vi "NI 9230 Getting Started (FPGA).vi"() -> ()   [LabVIEW 2021]
doc: "This VI acquires an arbitrary number of samples from each channel of the NI 9232 and places the acquired data into a DMA FIFO. The Input Configuration and Data Rate are configurable at run time."
uses:
  <vilib>/LabVIEW Targets/FPGA/cRIO/shared/nicrio_ModuleControls/nicrio_cRIO-9232_ConfigModeRing.ctl
  <vilib>/LabVIEW Targets/FPGA/cRIO/shared/nicrio_ModuleControls/nicrio_cRIO-9230_DataRatesRing2.ctl
  <vilib>/rvi/Emulation/niFpgaGetClockAttributes.vi
  <vilib>/rvi/Emulation/niFpgaSctlEmulationGetInTimedLoop.vi
  <vilib>/rvi/Emulation/niFpgaEmulationReportErrorSimple.vi
  <vilib>/rvi/eio/common/nirviEmuTemplatePropertySet_errors.vi
  <vilib>/rvi/eio/common/nirviEmuTemplateMethod_errors.vi
  <vilib>/rvi/interface/RandomDataEmulation/niFpgaRandomDataHandleErrors.vi
  <vilib>/rvi/Emulation/niFpgaCriticalErrorInLSC.vi
  <vilib>/eio/EIOPropertyNode/EIOPropertyNode.xnode
  <vilib>/eio/EIONode/EIONode.xnode
  <vilib>/rvi/DataTransferAndStorage/Container/XNode/niFpgaContainer.xnode
  <vilib>/rvi/interface/RandomDataEmulation/nirviRandomDataFpgaReadWriteTemplate.vi
  <vilib>/eio/EIOMethodNode/EIOMethodNode.xnode
  <vilib>/rvi/eio/common/nirviEmuTemplatePropertyGet_errors.vi
  <vilib>/rvi/eio/common/nirviEmuTemplatePropertyGet_noerrors.vi
  <vilib>/rvi/eio/common/nirviEmuTemplatePropertySet_noerrors.vi
panel:
  in  "Input Configuration 1":T1 items=["AC Coupled", "DC Coupled", "IEPE AC Coupled"]
  in  "Input Configuration 0":T1 items=["AC Coupled", "DC Coupled", "IEPE AC Coupled"]
  in  "Data Rate":T2=10 items=["12.800 kS/s (NI 9230)"=10, "11.378 kS/s (NI 9230)"=36, "10.240 kS/s (NI 9230)"=21, "9.309 kS/s (NI 9230)"=44, "8.533 kS/s (NI 9230)"=14, "7.877 kS/s (NI 9230)"=52, "7.314 kS/s (NI 9230)"=29, "6.827 kS/s (NI 9230)"=60, "6.400 kS/s (NI 9230)"=18, "6.024 kS/s (NI 9230)"=68, "5.689 kS/s (NI 9230)"=37, "5.389 kS/s (NI 9230)"=76, "5.120 kS/s (NI 9230)"=22, "4.876 kS/s (NI 9230)"=84, "4.655 kS/s (NI 9230)"=45, "4.452 kS/s (NI 9230)"=92, "4.267 kS/s (NI 9230)"=26, "4.096 kS/s (NI 9230)"=100, "3.938 kS/s (NI 9230)"=53, "3.657 kS/s (NI 9230)"=30, "3.413 kS/s (NI 9230)"=61, "3.200 kS/s (NI 9230)"=34, "3.012 kS/s (NI 9230)"=69, "2.844 kS/s (NI 9230)"=38, "2.695 kS/s (NI 9230)"=77, "2.560 kS/s (NI 9230)"=42, "2.438 kS/s (NI 9230)"=85, "2.327 kS/s (NI 9230)"=46, "2.226 kS/s (NI 9230)"=93, "2.133 kS/s (NI 9230)"=50, "2.048 kS/s (NI 9230)"=101, "1.969 kS/s (NI 9230)"=54, "1.829 kS/s (NI 9230)"=58, "1.707 kS/s (NI 9230)"=62, "1.600 kS/s (NI 9230)"=66, "1.506 kS/s (NI 9230)"=70, "1.422 kS/s (NI 9230)"=74, "1.347 kS/s (NI 9230)"=78, "1.280 kS/s (NI 9230)"=82, "1.219 kS/s (NI 9230)"=86, "1.164 kS/s (NI 9230)"=90, "1.113 kS/s (NI 9230)"=94, "1.067 kS/s (NI 9230)"=98, "1.024 kS/s (NI 9230)"=102, "0.985 kS/s (NI 9230)"=106]
  out "Error Out":errorcluster
  out "Short Circuit":bool[](array[boolean])
  out "Open Loop":bool[](array[boolean])
  in  "Input Configuration 2":T1 items=["AC Coupled", "DC Coupled", "IEPE AC Coupled"]
  out "Data FIFO Full":bool
  # "Overview: Demonstrates how to acquire data from the NI 9230\nRequirements: LabVIEW Full Development System, LV FPGA, and NI RIO\nInstructions: \n1. Run NI 9230 Getting Started (Host).vi"
  # "Input Parameters"
  # "Output Parameters"
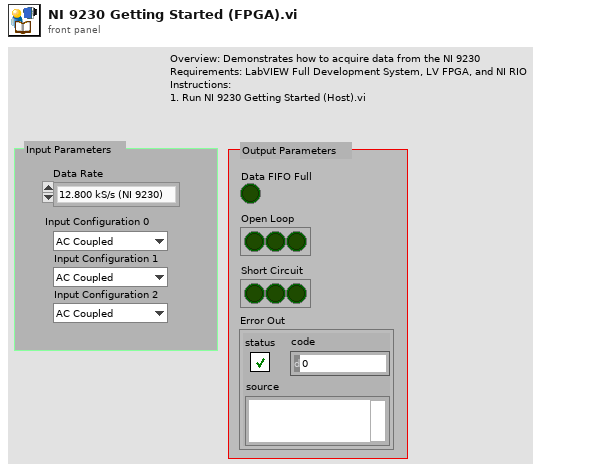
[diagram p1: front panel]
types:
  T1 = typedef "nicrio_cRIO-9232_ConfigModeRing.ctl" = u8
  T2 = typedef "nicrio_cRIO-9230_DataRatesRing2.ctl" = u8
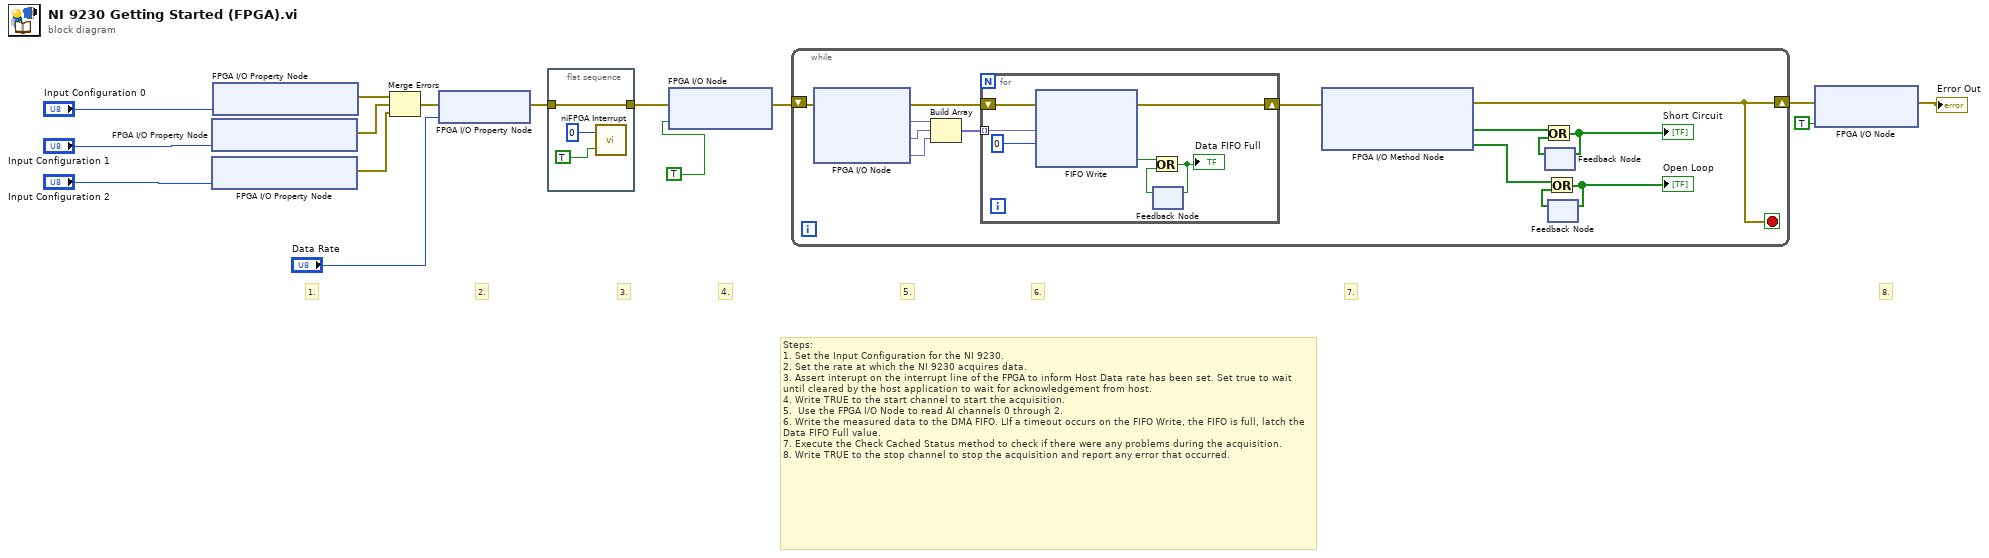
[diagram p0: block diagram]
diagram:
  # "5."
  # "8."
  # "7."
  # "Steps: \n1. Set the Input Configuration for the NI 9230.\n2. Set the rate at which the NI 9230 acquires data. \n3. Assert interupt on the interrupt line of the FPGA to inform Host Data rate has been set. Set true to wait until cleared by the host application to wait for acknowledgement from host.\n4. Write TRUE to the start channel to start the acquisition. \n5.  Use the FPGA I/O Node to read AI channels 0 through 2. \n6. Write the measured data to the DMA FIFO. LIf a timeout occurs on the FIFO Write, the FIFO is full, latch the Data FIFO Full value.\n7. Execute the Check Cached Status method to check if there were any problems during the acquisition.\n8. Write TRUE to the stop channel to stop the acquisition and report any error that occurred."
  # "6."
  # "4."
  # "2."
  # "3."
  # "1."
  n1 = xnode "FPGA I/O Property Node"("Input Configuration"="Input Configuration 1") -> ("error out"=w13:errorcluster)  [unwired: 2 in, 1 out]
  n2 = xnode "FPGA I/O Property Node"("Input Configuration"="Input Configuration 2") -> ("error out"=w12:errorcluster)  [unwired: 2 in, 1 out]
  n3 = xnode "FPGA I/O Property Node"("Input Configuration"="Input Configuration 0") -> ("error out"=w14:errorcluster)  [unwired: 2 in, 1 out]
  n4 = Merge Errors(w14, w13, w12) -> (w9:errorcluster)
  n5 = xnode "FPGA I/O Property Node"("error in"=w9, "Data Rate"="Data Rate") -> ("error out"=w11:errorcluster)  [unwired: 1 in, 1 out]
  n6 = flat-sequence {
    tunnel: [w16] -> w8
    tunnel: w11 -> [w16]
    frame #0 {
      n7 = call <vilib>:"niFPGA Interrupt.vi"("Wait Until Cleared (F)"=TRUE ("Wait Until Cleared"), "IRQ Number (0)"=u8 0 ("IRQ Bit (0-31)")) -> ()  [unwired: 1 in]
    }
  }
  n8 = xnode "FPGA I/O Node"("error in"=w8, "Mod3/Start"=TRUE) -> ("error out"=w6:errorcluster)  [unwired: 1 in, 1 out]
  n9 = while {
    shift-right: [w31] -> w5
    shift-left: w6 -> [w32]
    stop <- w31 stop-if-true
    n10 = xnode "FPGA I/O Node"("error in"=w32) -> ("error out"=w25:errorcluster, "Mod3/AI0"=w29:fxp<+/-,24,7>, "Mod3/AI1"=w28:fxp<+/-,24,7>, "Mod3/AI2"=w27:fxp<+/-,24,7>)  [unwired: 3 in, 3 out]
    n11 = Build Array(w29, w28, w27) -> (w26:fxp<+/-,24,7>[])
    n12 = for {
      tunnel: w26 -> [w36] mode=indexing
      shift-right: [w33] -> w30
      shift-left: w25 -> [w34]
      n13 = xnode ("FIFO Write")("Element"=w36, "Timeout"=0 ("Timeout (-1 for no timeout)"), "error in (no error)"=w34) -> ("Timed Out?"=w37:bool, "error out"=w33:errorcluster)  [unwired: 1 in, 1 out]
      n14 = feedback #1() -> (w38:bool)  [unwired: 1 out]
      n15 = Or(x=w37, y=w38) -> (x .or. y?=w39:bool)
      "Data FIFO Full" <- w39
      n16 = feedback-in #1(w39) -> ()
    }
    n17 = xnode "FPGA I/O Method Node"("error in"=w30) -> ("error out"=w31:errorcluster, "Short Circuit"=w20:bool[], "Open Loop"=w23:bool[])  [unwired: 1 in, 1 out]
    n18 = feedback #2() -> (w21:bool[])  [unwired: 1 out]
    n19 = Or(x=w20, y=w21) -> (x .or. y?=w19:bool[])
    "Short Circuit" <- w19
    n20 = feedback-in #2(w19) -> ()
    n21 = feedback #3() -> (w24:bool[])  [unwired: 1 out]
    n22 = Or(x=w23, y=w24) -> (x .or. y?=w22:bool[])
    "Open Loop" <- w22
    n23 = feedback-in #3(w22) -> ()
  }
  n24 = xnode "FPGA I/O Node"("error in"=w5, "Mod3/Stop"=TRUE) -> ("error out"=→"Error Out":errorcluster)  [unwired: 1 in, 1 out]
